vi "Auto Shoot Cube Command_wrapper.vi"(8 "Command Info In":T1, 11 "Shoot Cube Parameters":cluster{"Shot Preset":T4}) -> (0 "Command Info Out":T1)   [LabVIEW 2020]
uses:
  <vilib>/Rock Robotics/WPI/Framework/Command Status Info.ctl
  <vilib>/Rock Robotics/WPI/Framework/Completion Status.ctl
  <vilib>/Rock Robotics/WPI/Framework/Completion Notifier.ctl
  Implementation/Typedefs/Cube Shooting Presets.ctl
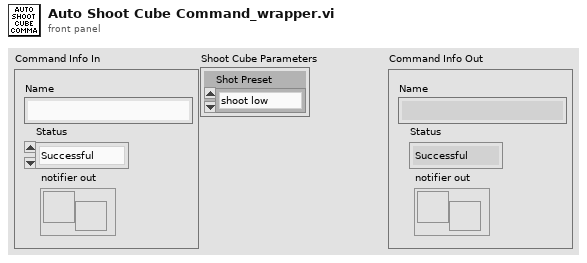
[diagram p1: front panel]
types:
  T1 = typedef "Command Status Info.ctl" = cluster{"Name":string, "Status":T2, "notifier out":T3}
  T2 = typedef "Completion Status.ctl" = enum16{"Successful", "Aborted", "Incomplete"}
  T3 = typedef "Completion Notifier.ctl" = refnum<notifier>
  T4 = typedef "Cube Shooting Presets.ctl" = enum16{"shoot low", "shoot mid", "shoot high"}
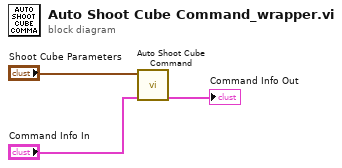
[diagram p0: block diagram]
diagram:
  n1 = call "Auto Shoot Cube Command.vi"("Command Info In"="Command Info In", "Shoot Cube Parameters"="Shoot Cube Parameters") -> ("Command Info Out"=→"Command Info Out":T1)  [unwired: 9 in]
